vi "CopyDataToGPU.vi"(0 "Array Src IN Host":u8[](array[numeric]), 4 "Error IN Toolkit":i32, 5 "Error IN LabVIEW":errorcluster) -> (18 "Error OUT LabVIEW":i32, 19 "Error OUT LabVIEW":errorcluster)   [LabVIEW 2018]
doc: "It copies a 1D U8 array stored in the CPU to the GPU and it returns an error code. It receives an array 1D U8 and an integer that will store the error.\nFor correct operation, you must pass the error that comes from the VI \"ReservationMemory\"."
uses:
  dll/LibreriaAutis_3.dll
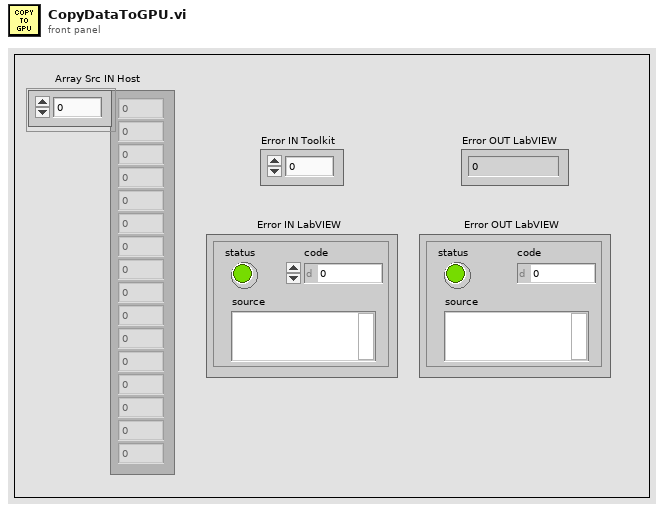
[diagram p1: front panel]
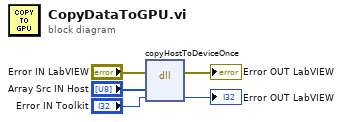
[diagram p0: block diagram]
diagram:
  n1 = dll-call lib="C:/Users/AUTIS/Desktop/LibreriaAUTIS/LabVIEW/dll/LibreriaAutis_3.dll" fn="copyHostToDeviceOnce"(error in="Error IN LabVIEW", "src"="Array Src IN Host", "error"="Error IN Toolkit") -> (error out=→"Error OUT LabVIEW":errorcluster, "error"=→"Error OUT LabVIEW":i32)  [unwired: 4 in, 1 out]
